vi "log analysis_gps.vi"() -> ()   [LabVIEW 2019] (continued)
\tsystem status\tnormal 2 27.900000 0 0\trobot status\t134.802859\t125.219329\t7.982200\t-2.716402\t-0.059958\t-178.151167\t0.301000\t-0.007000\n\t\n15:45:35.6\tlog_raw\tgps_raw\t#INSPVAXA,USB3,0,48.5,FINESTEERING,2107,283553.600,02000000,471d,15824;INS_ALIGNMENT_COMPLETE,INS_RTKFIXED,37.37125846696,126.72235533990,7.9816,22.3000,0.0235,-0.2652,0.0170,-2.709628745,-0.144831569,268.295218513,0.4383,0.2948,0.5739,0.1125,0.0924,0.0783,0.0963,0.1010,5.0842,0f000001,0*696fd9b1\n\tsystem status\tnormal 2 27.900000 0 0\trobot status\t134.659909\t125.219563\t7.981600\t-2.709629\t-0.144832\t-178.295219\t0.297000\t-0.009000\n\t\n15:45:36.1\tlog_raw\tgps_raw\t#DUALANTENNAHEADINGA,USB3,0,48.5,FINESTEERING,2107,283554.100,02000000,d426,15824;INSUFFICIENT_OBS,NONE,-1.000000000,0.000000000,0.000000000,0.0,0.000000000,0.000000000,\"631T\",13,4,4,3,04,00,20,02*de32c05b\n\tsystem status\tnormal 2 27.900000 0 0\trobot status\t134.520570\t125.219884\t7.981500\t-2.835282\t-0.233687\t-178.487489\t0.302000\t-0.003000\n\t\n15:45:36.6\tlog_raw\tgps_raw\t#INSPVAXA,USB3,0,51.0,FINESTEERING,2107,283554.600,02000000,471d,15824;INS_ALIGNMENT_COMPLETE,INS_RTKFIXED,37.37125848358,126.72235217781,7.9795,22.3000,0.0223,-0.2763,0.0124,-2.892819267,-0.280095971,268.699067349,0.4384,0.2951,0.5740,0.1126,0.0925,0.0783,0.0963,0.1010,5.0853,0f000001,0*82db867f\n\tsystem status\tnormal 2 27.900000 0 0\trobot status\t134.379816\t125.221412\t7.979500\t-2.892819\t-0.280096\t-178.699067\t0.295000\t-0.010000\n\t\n15:45:37.1\tlog_raw\tgps_raw\t#DUALANTENNAHEADINGA,USB3,0,47.0,FINESTEERING,2107,283555.100,02000000,d426,15824;INSUFFICIENT_OBS,NONE,-1.000000000,0.000000000,0.000000000,0.0,0.000000000,0.000000000,\"631T\",14,4,4,3,04,00,20,03*a9c2070c\n\tsystem status\tnormal 2 27.900000 0 0\trobot status\t134.235506\t125.223968\t7.977100\t-2.869099\t-0.294535\t-178.888664\t0.296000\t-0.003000\n\t\n15:45:37.6\tlog_raw\tgps_raw\t#INSPVAXA,USB3,0,47.0,FINESTEERING,2107,283555.600,02000000,471d,15824;INS_ALIGNMENT_COMPLETE,INS_RTKFIXED,37.37125853353,126.72234893237,7.9755,22.3000,0.0216,-0.2860,0.0144,-2.819506648,-0.407770491,269.082070244,0.4381,0.2951,0.5741,0.1126,0.0924,0.0783,0.0963,0.1010,5.0867,0f000001,0*4971d182\n\tsystem status\tnormal 2 27.900000 0 0\trobot status\t134.092341\t125.226961\t7.975500\t-2.819507\t-0.407770\t-179.082070\t0.300000\t-0.010000\n\t\n15:45:38.1\tlog_raw\tgps_raw\t#INSPVAXA,USB3,0,45.0,FINESTEERING,2107,283556.100,02000000,471d,15824;INS_ALIGNMENT_COMPLETE,INS_RTKFIXED,37.37125856914,126.72234737250,7.9744,22.3000,0.0229,-0.2921,0.0135,-2.758204349,-0.398675406,269.289539292,0.4378,0.2952,0.5740,0.1126,0.0924,0.0783,0.0962,0.1010,5.0883,0f000001,0*04f4864c\n\tsystem status\tnormal 2 27.900000 0 0\trobot status\t133.954170\t125.230915\t7.974400\t-2.758204\t-0.398675\t-179.289539\t0.302000\t-0.005000\n\t\n15:45:38.6\tlog_raw\tgps_raw\t#DUALANTENNAHEADINGA,USB3,0,45.0,FINESTEERING,2107,283556.600,02000000,d426,15824;INSUFFICIENT_OBS,NONE,-1.000000000,0.000000000,0.000000000,0.0,0.000000000,0.000000000,\"631T\",14,4,4,3,04,00,20,03*1b8bbdb9\n\tsystem status\tnormal 2 27.900000 0 0\trobot status\t133.810841\t125.235429\t7.973900\t-2.640531\t-0.361099\t-179.438538\t0.158000\t0.018000\n\t\n15:45:39.1\tlog_raw\tgps_raw\t#DUALANTENNAHEADINGA,USB3,0,45.0,FINESTEERING,2107,283557.100,02000000,d426,15824;INSUFFICIENT_OBS,NONE,-1.000000000,0.000000000,0.000000000,0.0,0.000000000,0.000000000,\"631T\",15,4,4,3,04,00,20,03*6d1923ae\n\tsystem status\tnormal 2 27.800000 0 0\trobot status\t133.723563\t125.240390\t7.973200\t-2.680477\t-0.214338\t-179.491663\t0.281000\t-0.012000\n\t\n15:45:39.6\tlog_raw\tgps_raw\t#DUALANTENNAHEADINGA,USB3,0,46.5,FINESTEERING,2107,283557.600,02000000,d426,15824;INSUFFICIENT_OBS,NONE,-1.000000000,0.000000000,0.000000000,0.0,0.000000000,0.000000000,\"631T\",14,4,4,3,04,00,20,03*8fe42440\n\tsystem status\tnormal 2 27.900000 0 0\trobot status\t133.557064\t125.247786\t7.971500\t-2.546712\t-0.382295\t-179.652165\t0.298000\t-0.007000\n\t\n15:45:40.1\tlog_raw\tgps_raw\t#DUALANTENNAHEADINGA,USB3,0,46.5,FINESTEERING,2107,283558.100,02000000,d426,15824;INSUFFICIENT_OBS,NONE,-1.000000000,0.000000000,0.000000000,0.0,0.000000000,0.000000000,\"631T\",11,4,4,3,04,00,20,02*089ab1fe\n\tsystem status\tnormal 2 27.900000 0 0\trobot status\t133.431382\t125.255378\t7.969700\t-2.437296\t-0.317017\t-179.816520\t0.288000\t-0.003000\n\t\n15:45:40.6\tlog_raw\tgps_raw\t#INSPVAXA,USB3,0,47.5,FINESTEERING,2107,283558.600,02000000,471d,15824;INS_ALIGNMENT_COMPLETE,INS_RTKFIXED,37.37125886562,126.72233975708,7.9685,22.3000,0.0526,-0.2759,0.0211,-2.409557071,-0.340107874,269.967780628,0.4378,0.2950,0.5739,0.1125,0.0924,0.0783,0.0962,0.1009,5.0913,0f000001,0*5e667246\n\tsystem status\tnormal 2 27.900000 0 0\trobot status\t133.279608\t125.263831\t7.968500\t-2.409557\t-0.340108\t-179.967781\t0.299000\t0.000000\n\t\n15:45:41.1\tlog_raw\tgps_raw\t#DUALANTENNAHEADINGA,USB3,0,47.5,FINESTEERING,2107,283559.100,02008000,d426,15824;INSUFFICIENT_OBS,NONE,-1.000000000,0.000000000,0.000000000,0.0,0.000000000,0.000000000,\"631T\",9,4,4,3,04,00,20,03*5bfaaf18\n\tsystem status\tnormal 2 27.900000 0 0\trobot status\t133.140609\t125.272278\t7.967700\t-2.441354\t-0.223495\t179.916297\t0.310000\t0.003000\n\t\n15:45:41.6\tlog_raw\tgps_raw\t#DUALANTENNAHEADINGA,USB3,0,51.0,FINESTEERING,2107,283559.600,02008000,d426,15824;INSUFFICIENT_OBS,NONE,-1.000000000,0.000000000,0.000000000,0.0,0.000000000,0.000000000,\"631T\",11,4,4,3,04,00,20,03*aa74f950\n\tsystem status\tnormal 2 27.900000 0 0\trobot status\t132.998565\t125.282342\t7.968400\t-2.323197\t-0.094957\t179.812330\t0.293000\t0.004000\n\t\n15:45:42.1\tlog_raw\tgps_raw\t#DUALANTENNAHEADINGA,USB3,0,43.5,FINESTEERING,2107,283560.100,02008000,d426,15824;INSUFFICIENT_OBS,NONE,-1.000000000,0.000000000,0.000000000,0.0,0.000000000,0.000000000,\"631T\",12,4,4,3,04,00,20,02*918dc314\n\tsystem status\tnormal 2 27.900000 0 0\trobot status\t132.851646\t125.293516\t7.969300\t-2.162737\t0.027270\t179.722426\t0.294000\t0.002000\n\t\n15:45:42.6\tlog_raw\tgps_raw\t#INSPVAXA,USB3,0,43.5,FINESTEERING,2107,283560.600,02008000,471d,15824;INS_ALIGNMENT_COMPLETE,INS_RTKFIXED,37.37125922477,126.72233331539,7.9711,22.3000,0.0461,-0.3029,0.0142,-2.105523961,0.098116504,270.318274292,0.4374,0.2952,0.5740,0.1125,0.0925,0.0783,0.0962,0.1009,5.0942,0f000001,0*4e7a44d6\n\tsystem status\tnormal 2 27.900000 0 0\trobot status\t132.709014\t125.303700\t7.971100\t-2.105524\t0.098117\t179.681726\t0.302000\t0.009000\n\t\n15:45:43.1\tlog_raw\tgps_raw\t\tsystem status\tnormal 2 27.900000 0 0\trobot status\t132.562472\t125.314678\t7.972700\t-2.092784\t0.038712\t179.551571\t0.231000\t0.029000\n\t\n15:45:43.6\tlog_raw\tgps_raw\t#DUALANTENNAHEADINGA,USB3,0,45.0,FINESTEERING,2107,283561.600,02008000,d426,15824;INSUFFICIENT_OBS,NONE,-1.000000000,0.000000000,0.000000000,0.0,0.000000000,0.000000000,\"631T\",11,4,4,3,04,00,20,03*333d7c31\n\tsystem status\tnormal 2 27.800000 0 0\trobot status\t132.438939\t125.326177\t7.973000\t-2.055838\t0.129600\t179.563628\t0.311000\t0.023000\n\t\n15:45:44.1\tlog_raw\tgps_raw\t#DUALANTENNAHEADINGA,USB3,0,45.0,FINESTEERING,2107,283562.100,02008000,d426,15824;INSUFFICIENT_OBS,NONE,-1.000000000,0.000000000,0.000000000,0.0,0.000000000,0.000000000,\"631T\",10,4,4,3,04,00,20,03*9e1feb94\n\tsystem status\tnormal 2 27.900000 0 0\trobot status\t132.286022\t125.338495\t7.973600\t-2.088322\t-0.039362\t179.462499\t0.292000\t0.007000\n\t\n15:45:44.6\tlog_raw\tgps_raw\t#DUALANTENNAHEADINGA,USB3,0,49.5,FINESTEERING,2107,283562.600,02008000,d426,15824;INSUFFICIENT_OBS,NONE,-1.000000000,0.000000000,0.000000000,0.0,0.000000000,0.000000000,\"631T\",11,4,4,3,04,00,20,03*0e8972e5\n\tsystem status\tnormal 2 27.900000 0 0\trobot status\t132.139609\t125.349583\t7.973900\t-2.147199\t-0.245096\t179.550470\t0.291000\t0.030000\n\t\n15:45:45.1\tlog_raw\tgps_raw\t#DUALANTENNAHEADINGA,USB3,0,49.5,FINESTEERING,2107,283563.100,02008000,d426,15824;INSUFFICIENT_OBS,NONE,-1.000000000,0.000000000,0.000000000,0.0,0.000000000,0.000000000,\"631T\",12,4,4,3,04,00,20,03*0cafea03\n\tsystem status\tnormal 2 27.800000 0 0\trobot status\t131.994665\t125.361643\t7.974000\t-2.066885\t-0.502356\t179.731447\t0.253000\t0.073000\n\t\n15:45:45.6\tlog_raw\tgps_raw\t#DUALANTENNAHEADINGA,USB3,0,49.5,FINESTEERING,2107,283563.600,02000000,d426,15824;INSUFFICIENT_OBS,NONE,-1.000000000,0.000000000,0.000000000,0.0,0.000000000,0.000000000,\"631T\",11,4,4,3,04,00,20,03*75c2f29d\n\tsystem status\tnormal 2 27.800000 0 0\trobot status\t131.850322\t125.373668\t7.974200\t-1.867187\t-0.627381\t-179.945539\t0.352000\t-0.066000\n\t\n15:45:46.1\tlog_raw\tgps_raw\t#DUALANTENNAHEADINGA,USB3,0,46.5,FINESTEERING,2107,283564.100,02000000,d426,15824;INSUFFICIENT_OBS,NONE,-1.000000000,0.000000000,0.000000000,0.0,0.000000000,0.000000000,\"631T\",12,4,4,3,04,00,20,03*b22ee873\n\tsystem status\tnormal 2 27.800000 0 0\trobot status\t131.705241\t125.384504\t7.975500\t-1.737840\t-0.783684\t-179.600630\t0.268000\t0.066000\n\t\n15:45:46.6\tlog_raw\tgps_raw\t#DUALANTENNAHEADINGA,USB3,0,46.5,FINESTEERING,2107,283564.600,02000000,d426,15824;INSUFFICIENT_OBS,NONE,-1.000000000,0.000000000,0.000000000,0.0,0.000000000,0.000000000,\"631T\",13,4,4,3,04,00,20,03*a96472bd\n\tsystem status\tnormal 2 27.700000 0 0\trobot status\t131.562793\t125.392691\t7.976300\t-1.793916\t-0.734413\t-179.145443\t0.390000\t-0.097000\n\t\n15:45:47.1\tlog_raw\tgps_raw\t#DUALANTENNAHEADINGA,USB3,0,46.5,FINESTEERING,2107,283565.100,02000000,d426,15824;INSUFFICIENT_OBS,NONE,-1.000000000,0.000000000,0.000000000,0.0,0.000000000,0.000000000,\"631T\",13,4,4,3,04,00,20,03*08146cf2\n\tsystem status\tnormal 2 27.700000 0 0\trobot status\t131.420891\t125.399247\t7.976000\t-1.910475\t-0.662509\t-178.628817\t0.261000\t0.086000\n\t\n15:45:47.6\tlog_raw\tgps_raw\t#DUALANTENNAHEADINGA,USB3,0,48.0,FINESTEERING,2107,283565.600,02000000,d426,15824;INSUFFICIENT_OBS,NONE,-1.000000000,0.000000000,0.000000000,0.0,0.000000000,0.000000000,\"631T\",12,4,4,3,04,00,20,03*500b58cb\n\tsystem status\tnormal 2 27.700000 0 0\trobot status\t131.278267\t125.405143\t7.974600\t-1.874953\t-0.506860\t-178.110215\t0.404000\t-0.126000\n\t\n15:45:48.1\tlog_raw\tgps_raw\t#DUALANTENNAHEADINGA,USB3,0,48.0,FINESTEERING,2107,283566.100,02000000,d426,15824;INSUFFICIENT_OBS,NONE,-1.000000000,0.000000000,0.000000000,0.0,0.000000000,0.000000000,\"631T\",13,4,4,3,04,00,20,02*8a2efff8\n\tsystem status\tnormal 2 27.700000 0 0\trobot status\t131.149443\t125.410077\t7.973900\t-1.835673\t-0.302067\t-177.605096\t0.432000\t-0.159000\n\t\n15:45:48.6\tlog_raw\tgps_raw\t\tsystem status\tnormal 2 27.700000 0 0\trobot status\t131.007001\t125.413685\t7.975600\t-1.683560\t-0.282934\t-177.105716\t0.327000\t-0.010000\n\t\n15:45:49.1\tlog_raw\tgps_raw\t#INSPVAXA,USB3,0,47.0,FINESTEERING,2107,283567.150,02000000,471d,15824;INS_ALIGNMENT_COMPLETE,INS_RTKFIXED,37.37126023924,126.72231232835,7.9766,22.3000,0.0196,-0.2915,0.0203,-1.615683840,-0.184237550,266.738571120,0.4436,0.2960,0.5749,0.1133,0.0925,0.0784,0.0962,0.1011,5.1038,0f000001,0*2b446319\n\tsystem status\tnormal 2 27.700000 0 0\trobot status\t130.850016\t125.416320\t7.976600\t-1.615684\t-0.184238\t-176.738571\t0.310000\t-0.001000\n\t\n15:45:49.6\tlog_raw\tgps_raw\t#DUALANTENNAHEADINGA,USB3,0,47.0,FINESTEERING,2107,283567.600,02000000,d426,15824;INSUFFICIENT_OBS,NONE,-1.000000000,0.000000000,0.000000000,0.0,0.000000000,0.000000000,\"631T\",12,4,4,3,04,00,20,02*8ed7ff70\n\tsystem status\tnormal 2 27.800000 0 0\trobot status\t130.720508\t125.417185\t7.976700\t-1.694653\t-0.119094\t-176.472297\t0.377000\t-0.106000\n\t\n15:45:50.1\tlog_raw\tgps_raw\t#DUALANTENNAHEADINGA,USB3,0,47.0,FINESTEERING,2107,283568.100,02000000,d426,15824;INSUFFICIENT_OBS,NONE,-1.000000000,0.000000000,0.000000000,0.0,0.000000000,0.000000000,\"631T\",14,4,4,3,04,00,20,03*aaffec67\n\tsystem status\tnormal 2 27.800000 0 0\trobot status\t130.578522\t125.417897\t7.977700\t-1.786957\t0.019040\t-176.223413\t0.280000\t0.039000\n\t\n15:45:50.6\tlog_raw\tgps_raw\t#INSPVAXA,USB3,0,50.5,FINESTEERING,2107,283568.650,02000000,471d,15824;INS_ALIGNMENT_COMPLETE,INS_RTKFIXED,37.37126026613,126.72230748127,7.9785,22.3000,0.0314,-0.2890,0.0136,-1.676303872,0.031387209,266.013991723,0.4441,0.2961,0.5750,0.1133,0.0925,0.0784,0.0962,0.1011,5.1051,0f000001,0*382c449f\n\tsystem status\tnormal 2 27.800000 0 0\trobot status\t130.420670\t125.419311\t7.978500\t-1.676304\t0.031387\t-176.013992\t0.335000\t-0.037000\n\t\n15:45:51.1\tlog_raw\tgps_raw\t#DUALANTENNAHEADINGA,USB3,0,40.0,FINESTEERING,2107,283569.100,02000000,d426,15824;INSUFFICIENT_OBS,NONE,-1.000000000,0.000000000,0.000000000,0.0,0.000000000,0.000000000,\"631T\",13,4,4,3,04,00,20,02*1cb1745e\n\tsystem status\tnormal 2 27.800000 0 0\trobot status\t130.289708\t125.420071\t7.978300\t-1.557732\t0.003070\t-175.975563\t0.340000\t-0.063000\n\t\n15:45:51.6\tlog_raw\tgps_raw\t#DUALANTENNAHEADINGA,USB3,0,40.0,FINESTEERING,2107,283569.600,02000000,d426,15824;INSUFFICIENT_OBS,NONE,-1.000000000,0.000000000,0.000000000,0.0,0.000000000,0.000000000,\"631T\",13,4,4,3,04,00,20,03*a71e5e5e\n\tsystem status\tnormal 2 27.800000 0 0\trobot status\t130.146113\t125.419852\t7.978500\t-1.454637\t0.095316\t-175.896222\t0.295000\t0.006000\n\t\n15:45:52.1\tlog_raw\tgps_raw\t#INSPVAXA,USB3,0,51.0,FINESTEERING,2107,283570.150,02000000,471d,15824;INS_ALIGNMENT_COMPLETE,INS_RTKFIXED,37.37126027188,126.72230260848,7.9782,22.3000,0.0223,-0.2985,0.0040,-1.310118648,0.027956781,265.914374243,0.4449,0.2965,0.5753,0.1133,0.0927,0.0784,0.0962,0.1011,5.1080,0f000001,0*e4cc9c92\n\tsystem status\tnormal 2 27.800000 0 0\trobot status\t129.989046\t125.419956\t7.978200\t-1.310119\t0.027957\t-175.914374\t0.293000\t0.021000\n\t\n15:45:52.6\tlog_raw\tgps_raw\t#INSPVAXA,USB3,0,51.0,FINESTEERING,2107,283570.650,02000000,471d,15824;INS_ALIGNMENT_COMPLETE,INS_RTKFIXED,37.37126026750,126.72230111428,7.9776,22.3000,0.0310,-0.1470,0.0080,-1.255276150,-0.174138807,265.875286689,0.4449,0.2965,0.5753,0.1133,0.0927,0.0784,0.0962,0.1011,5.1080,0f000001,0*fb01e8e4\n\tsystem status\tnormal 2 27.900000 0 0\trobot status\t129.856693\t125.419472\t7.977600\t-1.255276\t-0.174139\t-175.875287\t0.139000\t0.065000\n\t\n15:45:53.1\tlog_raw\tgps_raw\t#INSPVAXA,USB3,0,50.0,FINESTEERING,2107,283571.150,02000000,471d,15824;INS_ALIGNMENT_COMPLETE,INS_RTKFIXED,37.37126027111,126.72229951558,7.9776,22.3000,-0.0095,-0.3504,-0.0012,-1.130419534,-0.185484043,265.929537810,0.4449,0.2965,0.5753,0.1133,0.0927,0.0784,0.0962,0.1011,5.1080,0f000001,0*20782363\n\tsystem status\tnormal 2 27.800000 0 0\trobot status\t129.715082\t125.419874\t7.977600\t-1.130420\t-0.185484\t-175.929538\t0.366000\t-0.034000\n\t\n15:45:53.6\tlog_raw\tgps_raw\t\tsystem status\tnormal 2 27.800000 0 0\trobot status\t129.601866\t125.425975\t7.981400\t-0.935962\t-0.226185\t-175.828479\t0.305000\t0.000000\n\t\n15:45:54.1\tlog_raw\tgps_raw\t#DUALANTENNAHEADINGA,USB3,0,50.0,FINESTEERING,2107,283572.100,02000000,d426,15824;INSUFFICIENT_OBS,NONE,0.000000000,0.000000000,0.000000000,0.0,0.000000000,0.000000000,\"\",0,0,0,0,00,00,00,00*5d8535fc\n\tsystem status\tnormal 2 27.900000 0 0\trobot status\t129.452172\t125.430719\t7.986500\t-0.803584\t-0.452987\t-175.991155\t0.278000\t-0.004000\n\t\n15:45:54.6\tlog_raw\tgps_raw\t#DUALANTENNAHEADINGA,USB3,0,52.5,FINESTEERING,2107,283572.600,02000000,d426,15824;INSUFFICIENT_OBS,NONE,0.000000000,0.000000000,0.000000000,0.0,0.000000000,0.000000000,\"\",0,0,0,0,00,00,00,00*859f07a2\n\tsystem status\tnormal 2 27.900000 0 0\trobot status\t129.304513\t125.435695\t7.990800\t-0.754578\t-0.513148\t-176.084037\t0.303000\t-0.001000\n\t\n15:45:55.1\tlog_raw\tgps_raw\t#DUALANTENNAHEADINGA,USB3,0,50.0,FINESTEERING,2107,283573.100,02000000,d426,15824;INSUFFICIENT_OBS,NONE,0.000000000,0.000000000,0.000000000,0.0,0.000000000,0.000000000,\"\",0,0,0,0,00,00,00,00*a797c2ea\n\tsystem status\tnormal 2 27.900000 0 0\trobot status\t129.165268\t125.438398\t7.993900\t-0.825963\t-0.339685\t-176.124396\t0.304000\t0.001000\n\t\n15:45:55.6\tlog_raw\tgps_raw\t\tsystem status\tnormal 2 27.900000 0 0\trobot status\t129.021483\t125.428571\t7.991000\t-0.801949\t-0.273048\t-176.197065\t0.293000\t-0.010000\n\t\n15:45:56.1\tlog_raw\tgps_raw\t\tsystem status\tnormal 2 27.900000 0 0\trobot status\t128.872499\t125.421188\t7.988200\t-0.569716\t-0.162658\t-176.307146\t0.297000\t-0.004000\n\t\n15:45:56.6\tlog_raw\tgps_raw\t#INSPVAXA,USB3,0,52.0,FINESTEERING,2107,283574.650,02000000,471d,15824;INS_ALIGNMENT_COMPLETE,INS_RTKFIXED,37.37126025479,126.72228822591,7.9861,22.3000,0.0090,-0.3026,-0.0003,-0.524199220,-0.126443269,266.389234836,0.4991,0.3317,0.6500,0.1205,0.0986,0.0804,0.0985,0.1030,5.1132,0f000001,0*c3c99d89\n\tsystem status\tnormal 2 27.900000 0 0\trobot status\t128.715062\t125.418079\t7.986100\t-0.524199\t-0.126443\t-176.389235\t0.303000\t-0.004000\n\t\n15:45:57.1\tlog_raw\tgps_raw\t#INSPVAXA,USB3,0,50.0,FINESTEERING,2107,283575.150,02000000,471d,15824;INS_ALIGNMENT_COMPLETE,INS_RTKFIXED,37.37126023129,126.72228662486,7.9852,22.3000,0.0085,-0.2932,0.0017,-0.596688743,-0.097225443,266.485321234,0.4751,0.3142,0.6322,0.1185,0.0977,0.0789,0.0982,0.1027,5.1147,0f000001,0*e174b094\n\tsystem status\tnormal 2 27.900000 0 0\trobot status\t128.573243\t125.415473\t7.985200\t-0.596689\t-0.097225\t-176.485321\t0.297000\t-0.011000\n\t\n15:45:57.6\tlog_raw\tgps_raw\t#INSPVAXA,USB3,0,50.0,FINESTEERING,2107,283575.650,02000000,471d,15824;INS_ALIGNMENT_COMPLETE,INS_RTKFIXED,37.37126022571,126.72228518067,7.9842,22.3000,-0.0010,-0.2887,0.0210,-0.683424263,-0.147084143,266.527685008,0.4751,0.3142,0.6322,0.1185,0.0977,0.0789,0.0982,0.1027,5.1147,0f000001,0*c2e268d1\n\tsystem status\tnormal 2 27.900000 0 0\trobot status\t128.445319\t125.414855\t7.984200\t-0.683424\t-0.147084\t-176.527685\t0.295000\t-0.014000\n\t\n15:45:58.1\tlog_raw\tgps_raw\t#INSPVAXA,USB3,0,50.0,FINESTEERING,2107,283576.150,02000000,471d,15824;INS_ALIGNMENT_COMPLETE,INS_RTKFIXED,37.37126021633,126.72228346240,7.9840,22.3000,0.0021,-0.2751,0.0114,-0.667866815,-0.315367181,266.708831075,0.4606,0.3053,0.6179,0.1181,0.0979,0.0781,0.0979,0.1024,5.1163,0f000001,0*0ba78e3d\n\tsystem status\tnormal 2 27.900000 0 0\trobot status\t128.293118\t125.413817\t7.984000\t-0.667867\t-0.315367\t-176.708831\t0.298000\t-0.010000\n\t\n15:45:58.6\tlog_raw\tgps_raw\t#INSPVAXA,USB3,0,50.0,FINESTEERING,2107,283576.650,02000000,471d,15824;INS_ALIGNMENT_COMPLETE,INS_RTKFIXED,37.37126022512,126.72228190722,7.9848,22.3000,-0.0006,-0.2994,0.0229,-0.670999350,-0.155338039,266.786409078,0.4606,0.3053,0.6179,0.1181,0.0979,0.0781,0.0979,0.1024,5.1163,0f000001,0*9811c325\n\tsystem status\tnormal 2 27.900000 0 0\trobot status\t128.155363\t125.414794\t7.984800\t-0.670999\t-0.155338\t-176.786409\t0.310000\t-0.008000\n\t\n15:45:59.1\tlog_raw\tgps_raw\t\tsystem status\tnormal 2 27.900000 0 0\trobot status\t128.030138\t125.416182\t7.985200\t-0.637257\t-0.102027\t-176.886811\t0.297000\t-0.010000\n\t\n15:45:59.6\tlog_raw\tgps_raw\t#INSPVAXA,USB3,0,48.5,FINESTEERING,2107,283577.650,02000000,471d,15824;INS_ALIGNMENT_COMPLETE,INS_RTKFIXED,37.37126026454,126.72227868899,7.9856,22.3000,0.0080,-0.2785,0.0173,-0.609374053,-0.154098562,267.060666338,0.4521,0.3012,0.6064,0.1181,0.0980,0.0776,0.0975,0.1023,5.1178,0f000001,0*aa9c2bc5\n\tsystem status\tnormal 2 27.900000 0 0\trobot status\t127.870297\t125.419174\t7.985600\t-0.609374\t-0.154099\t-177.060666\t0.297000\t-0.010000\n\t\n15:46:00.1\tlog_raw\tgps_raw\t\tsystem status\tnormal 2 27.900000 0 0\trobot status\t127.740454\t125.423243\t7.986100\t-0.487780\t-0.129325\t-177.210178\t0.305000\t-0.013000\n\t\n15:46:00.6\tlog_raw\tgps_raw\t\tsystem status\tnormal 2 27.900000 0 0\trobot status\t127.598271\t125.426877\t7.987900\t-0.577346\t-0.157853\t-177.428203\t0.301000\t-0.011000\n\t\n15:46:01.1\tlog_raw\tgps_raw\t#INSPVAXA,USB3,0,51.5,FINESTEERING,2107,283579.150,02000000,471d,15824;INS_ALIGNMENT_COMPLETE,INS_RTKFIXED,37.37126037410,126.72227378516,7.9904,22.3000,0.0163,-0.2830,0.0173,-0.746603441,-0.380752059,267.626447850,0.4463,0.2992,0.5904,0.1180,0.0971,0.0775,0.0966,0.1018,5.1209,0f000001,0*da9a51df\n\tsystem status\tnormal 2 27.900000 0 0\trobot status\t127.435924\t125.431340\t7.990400\t-0.746603\t-0.380752\t-177.626448\t0.295000\t0.002000\n\t\n15:46:01.6\tlog_raw\tgps_raw\t#INSPVAXA,USB3,0,51.5,FINESTEERING,2107,283579.650,02000000,471d,15824;INS_ALIGNMENT_COMPLETE,INS_RTKFIXED,37.37126042399,126.72227213267,7.9925,22.3000,0.0129,-0.2940,0.0192,-0.723337751,-0.333271037,267.787526970,0.4463,0.2992,0.5904,0.1180,0.0971,0.0775,0.0966,0.1018,5.1209,0f000001,0*2d4308ff\n\tsystem status\tnormal 2 27.900000 0 0\trobot status\t127.289549\t125.436879\t7.992500\t-0.723338\t-0.333271\t-177.787527\t0.298000\t-0.005000\n\t\n15:46:02.1\tlog_raw\tgps_raw\t#INSPVAXA,USB3,0,52.5,FINESTEERING,2107,283580.150,02000000,471d,15824;INS_ALIGNMENT_COMPLETE,INS_RTKFIXED,37.37126049043,126.72227055501,7.9950,22.3000,0.0243,-0.3033,0.0180,-0.573377117,-0.330323438,267.951447700,0.4448,0.2989,0.5852,0.1175,0.0961,0.0776,0.0961,0.1014,5.1224,0f000001,0*65285ec1\n\tsystem status\tnormal 2 27.900000 0 0\trobot status\t127.149802\t125.444255\t7.995000\t-0.573377\t-0.330323\t-177.951448\t0.300000\t-0.003000\n\t\n15:46:02.6\tlog_raw\tgps_raw\t\tsystem status\tnormal 2 27.900000 0 0\trobot status\t127.021740\t125.451168\t7.997000\t-0.486595\t-0.381728\t-178.092435\t0.295000\t-0.004000\n\t\n15:46:03.1\tlog_raw\tgps_raw\t#DUALANTENNAHEADINGA,USB3,0,48.0,FINESTEERING,2107,283581.100,02000000,d426,15824;INSUFFICIENT_OBS,NONE,0.000000000,0.000000000,0.000000000,0.0,0.000000000,0.000000000,\"\",0,0,0,0,00,00,00,00*0d472a41\n\tsystem status\tnormal 2 27.900000 0 0\trobot status\t126.878207\t125.458703\t7.999100\t-0.601198\t-0.320020\t-178.256056\t0.297000\t0.000000\n\t\n15:46:03.6\tlog_raw\tgps_raw\t#INSPVAXA,USB3,0,48.0,FINESTEERING,2107,283581.650,02000000,471d,15824;INS_ALIGNMENT_COMPLETE,INS_RTKFIXED,37.37126070396,126.72226577509,8.0028,22.3000,0.0230,-0.2933,0.0344,-0.578760971,-0.170041590,268.380757067,0.4441,0.2986,0.5812,0.1168,0.0951,0.0777,0.0958,0.1011,5.1238,0f000001,0*94c5c4b2\n\tsystem status\tnormal 2 27.900000 0 0\trobot status\t126.726405\t125.467960\t8.002800\t-0.578761\t-0.170042\t-178.380757\t0.306000\t-0.001000\n\t\n15:46:04.1\tlog_raw\tgps_raw\t\tsystem status\tnormal 2 27.900000 0 0\trobot status\t126.600259\t125.475820\t8.006300\t-0.540708\t-0.165891\t-178.462661\t0.304000\t0.009000\n\t\n15:46:04.6\tlog_raw\tgps_raw\t#INSPVAXA,USB3,0,50.0,FINESTEERING,2107,283582.650,02000000,471d,15824;INS_ALIGNMENT_COMPLETE,INS_RTKFIXED,37.37126086300,126.72226255094,8.0114,22.3000,0.0186,-0.2902,0.0297,-0.554451124,-0.113657827,268.567093928,0.4437,0.2982,0.5783,0.1160,0.0941,0.0779,0.0956,0.1009,5.1252,0f000001,0*de1d38ac\n\tsystem status\tnormal 2 27.900000 0 0\trobot status\t126.440815\t125.485615\t8.011400\t-0.554451\t-0.113658\t-178.567094\t0.299000\t0.008000\n\t\n15:46:05.1\tlog_raw\tgps_raw\t#INSPVAXA,USB3,0,52.0,FINESTEERING,2107,283583.150,02000000,471d,15824;INS_ALIGNMENT_COMPLETE,INS_RTKFIXED,37.37126094107,126.72226089314,8.0147,22.3000,0.0176,-0.2816,0.0224,-0.681553326,-0.108375043,268.657687253,0.4431,0.2976,0.5763,0.1151,0.0933,0.0781,0.0955,0.1007,5.1266,0f000001,0*8a630b8d\n\tsystem status\tnormal 2 27.900000 0 0\trobot status\t126.293970\t125.494282\t8.014700\t-0.681553\t-0.108375\t-178.657687\t0.297000\t0.007000\n\t\n15:46:05.6\tlog_raw\tgps_raw\t#INSPVAXA,USB3,0,52.0,FINESTEERING,2107,283583.650,02000000,471d,15824;INS_ALIGNMENT_COMPLETE,INS_RTKFIXED,37.37126102705,126.72225926038,8.0174,22.3000,0.0194,-0.3033,0.0147,-0.616207417,-0.286762817,268.672715403,0.4431,0.2976,0.5763,0.1151,0.0933,0.0781,0.0955,0.1007,5.1266,0f000001,0*61848793\n\tsystem status\tnormal 2 27.900000 0 0\trobot status\t126.149343\t125.503827\t8.017400\t-0.616207\t-0.286763\t-178.672715\t0.308000\t0.006000\n\t\n15:46:06.1\tlog_raw\tgps_raw\t#INSPVAXA,USB3,0,52.0,FINESTEERING,2107,283584.150,02000000,471d,15824;INS_ALIGNMENT_COMPLETE,INS_RTKFIXED,37.37126112105,126.72225762489,8.0208,22.3000,0.0251,-0.2868,0.0143,-0.484996115,-0.348090113,268.682050647,0.4426,0.2969,0.5750,0.1144,0.0927,0.0782,0.0955,0.1006,5.1279,0f000001,0*d30f3e54\n\tsystem status\tnormal 2 27.900000 0 0\trobot status\t126.004474\t125.514261\t8.020800\t-0.484996\t-0.348090\t-178.682051\t0.301000\t0.006000\n\t\n15:46:06.6\tlog_raw\tgps_raw\t#INSPVAXA,USB3,0,52.0,FINESTEERING,2107,283584.650,02000000,471d,15824;INS_ALIGNMENT_COMPLETE,INS_RTKFIXED,37.37126121621,126.72225620166,8.0227,22.3000,0.0321,-0.0816,0.0199,-0.459149355,-0.498683965,268.628376377,0.4426,0.2969,0.5750,0.1144,0.0927,0.0782,0.0955,0.1006,5.1279,0f000001,0*e5ed7c63\n\tsystem status\tnormal 2 27.900000 0 0\trobot status\t125.878406\t125.524825\t8.022700\t-0.459149\t-0.498684\t-178.628376\t0.142000\t0.011000\n\t\n15:46:07.1\tlog_raw\tgps_raw\t#INSPVAXA,USB3,0,49.0,FINESTEERING,2107,283585.150,02000000,471d,15824;INS_ALIGNMENT_COMPLETE,INS_RTKFIXED,37.37126129698,126.72225459849,8.0251,22.3000,0.0349,-0.3426,0.0329,-0.569349800,-0.560640511,268.532383253,0.4425,0.2966,0.5744,0.1144,0.0924,0.0784,0.0956,0.1006,5.1294,0f000001,0*4640cbf6\n\tsystem status\tnormal 2 27.700000 0 0\trobot status\t125.736400\t125.533791\t8.025100\t-0.569350\t-0.560641\t-178.532383\t0.389000\t-0.081000\n\t\n15:46:07.6\tlog_raw\tgps_raw\t#INSPVAXA,USB3,0,49.0,FINESTEERING,2107,283585.650,02000000,471d,15824;INS_ALIGNMENT_COMPLETE,INS_RTKFIXED,37.37126137394,126.72225308543,8.0277,22.3000,0.0305,-0.3477,0.0168,-0.707352535,-0.516144165,268.333596331,0.4425,0.2966,0.5744,0.1144,0.0924,0.0784,0.0956,0.1006,5.1294,0f000001,0*ea5ffab2\n\tsystem status\tnormal 2 27.800000 0 0\trobot status\t125.602376\t125.542334\t8.027700\t-0.707353\t-0.516144\t-178.333596\t0.335000\t0.002000\n\t\n15:46:08.1\tlog_raw\tgps_raw\t#INSPVAXA,USB3,0,50.5,FINESTEERING,2107,283586.150,02000000,471d,15824;INS_ALIGNMENT_COMPLETE,INS_RTKFIXED,37.37126146482,126.72225147889,8.0290,22.3000,0.0318,-0.3117,0.0162,-0.540726540,-0.516678625,268.023762114,0.4406,0.2960,0.5741,0.1134,0.0922,0.0785,0.0957,0.1006,5.1306,0f000001,0*2ae37417\n\tsystem status\tnormal 2 27.800000 0 0\trobot status\t125.460071\t125.552423\t8.029000\t-0.540727\t-0.516679\t-178.023762\t0.289000\t0.030000\n\t\n15:46:08.6\tlog_raw\tgps_raw\t#INSPVAXA,USB3,0,50.5,FINESTEERING,2107,283586.650,02000000,471d,15824;INS_ALIGNMENT_COMPLETE,INS_RTKFIXED,37.37126154442,126.72224983237,8.0302,22.3000,0.0153,-0.2976,0.0132,-0.405221817,-0.801510438,267.749524136,0.4406,0.2960,0.5741,0.1134,0.0922,0.0785,0.0957,0.1006,5.1306,0f000001,0*889b905c\n\tsystem status\tnormal 2 27.800000 0 0\trobot status\t125.314225\t125.561259\t8.030200\t-0.405222\t-0.801510\t-177.749524\t0.329000\t-0.031000\n\t\n15:46:09.1\tlog_raw\tgps_raw\t#INSPVAXA,USB3,0,48.5,FINESTEERING,2107,283587.150,02000000,471d,15824;INS_ALIGNMENT_COMPLETE,INS_RTKFIXED,37.37126161078,126.72224818389,8.0314,22.3000,0.0135,-0.2861,0.0058,-0.357423684,-1.016170306,267.360005702,0.4401,0.2956,0.5740,0.1128,0.0921,0.0786,0.0958,0.1006,5.1321,0f000001,0*b354eb89\n\tsystem status\tnormal 2 27.700000 0 0\trobot status\t125.168205\t125.568626\t8.031400\t-0.357424\t-1.016170\t-177.360006\t0.215000\t0.133000\n\t\n15:46:09.6\tlog_raw\tgps_raw\t#DUALANTENNAHEADINGA,USB3,0,48.5,FINESTEERING,2107,283587.600,02000000,d426,15824;INSUFFICIENT_OBS,NONE,0.000000000,0.000000000,0.000000000,0.0,0.000000000,0.000000000,\"\",0,0,0,0,00,00,00,00*3e024a6f\n\tsystem status\tnormal 2 27.700000 0 0\trobot status\t125.039123\t125.573448\t8.032800\t-0.358744\t-1.223027\t-176.913005\t0.232000\t0.115000\n\t\n15:46:10.1\tlog_raw\tgps_raw\t\tsystem status\tnormal 2 27.700000 0 0\trobot status\t124.894346\t125.578707\t8.033000\t-0.333259\t-1.304373\t-176.475504\t0.206000\t0.158000\n\t\n15:46:10.6\tlog_raw\tgps_raw\t#INSPVAXA,USB3,0,49.5,FINESTEERING,2107,283588.650,02000000,471d,15824;INS_ALIGNMENT_COMPLETE,INS_RTKFIXED,37.37126174157,126.72224330005,8.0321,22.3000,0.0403,-0.2838,0.0098,-0.134470490,-1.230467800,265.991496419,0.4395,0.2955,0.5741,0.1126,0.0921,0.0786,0.0959,0.1007,5.1336,0f000001,0*86c47da8\n\tsystem status\tnormal 2 27.700000 0 0\trobot status\t124.735603\t125.583149\t8.032100\t-0.134470\t-1.230468\t-175.991496\t0.276000\t0.046000\n\t\n15:46:11.1\tlog_raw\tgps_raw\t#INSPVAXA,USB3,0,51.5,FINESTEERING,2107,283589.150,02000000,471d,15824;INS_ALIGNMENT_COMPLETE,INS_RTKFIXED,37.37126177483,126.72224169465,8.0328,22.3000,0.0428,-0.2922,0.0200,-0.044724950,-0.991745549,265.567471181,0.4384,0.2954,0.5742,0.1124,0.0922,0.0786,0.0960,0.1008,5.1352,0f000001,0*fd2974d4\n\tsystem status\tnormal 2 27.700000 0 0\trobot status\t124.593399\t125.586842\t8.032800\t-0.044725\t-0.991746\t-175.567471\t0.295000\t0.021000\n\t\n15:46:11.6\tlog_raw\tgps_raw\t#INSPVAXA,USB3,0,51.5,FINESTEERING,2107,283589.650,02000000,471d,15824;INS_ALIGNMENT_COMPLETE,INS_RTKFIXED,37.37126179570,126.72224014857,8.0325,22.3000,0.0430,-0.3072,0.0249,-0.007617366,-0.680507333,265.196792969,0.4384,0.2954,0.5742,0.1124,0.0922,0.0786,0.0960,0.1008,5.1352,0f000001,0*75474069\n\tsystem status\tnormal 2 27.700000 0 0\trobot status\t124.456450\t125.589160\t8.032500\t-0.007617\t-0.680507\t-175.196793\t0.366000\t-0.059000\n\t\n15:46:12.1\tlog_raw\tgps_raw\t#INSPVAXA,USB3,0,52.0,FINESTEERING,2107,283590.150,02000000,471d,15824;INS_ALIGNMENT_COMPLETE,INS_RTKFIXED,37.37126181306,126.72223852203,8.0321,22.3000,0.0371,-0.3064,0.0221,-0.054866167,-0.319461022,264.939008114,0.4379,0.2954,0.5744,0.1124,0.0922,0.0786,0.0960,0.1008,5.1368,0f000001,0*489db8a8\n\tsystem status\tnormal 2 27.800000 0 0\trobot status\t124.312374\t125.591089\t8.032100\t-0.054866\t-0.319461\t-174.939008\t0.268000\t0.071000\n\t\n15:46:12.6\tlog_raw\tgps_raw\t#INSPVAXA,USB3,0,52.0,FINESTEERING,2107,283590.650,02000000,471d,15824;INS_ALIGNMENT_COMPLETE,INS_RTKFIXED,37.37126182845,126.72223689511,8.0304,22.3000,0.0329,-0.2983,0.0263,-0.099615260,-0.144209123,264.670119268,0.4379,0.2954,0.5744,0.1124,0.0922,0.0786,0.0960,0.1008,5.1368,0f000001,0*3ff0cb58\n\tsystem status\tnormal 2 27.800000 0 0\trobot status\t124.168264\t125.592799\t8.030400\t-0.099615\t-0.144209\t-174.670119\t0.312000\t-0.012000\n\t\n15:46:13.1\tlog_raw\tgps_raw\t\tsystem status\tnormal 2 27.800000 0 0\trobot status\t124.023646\t125.595225\t8.029500\t-0.060509\t-0.092324\t-174.506927\t0.241000\t0.080000\n\t\n15:46:13.6\tlog_raw\tgps_raw\t#INSPVAXA,USB3,0,46.5,FINESTEERING,2107,283591.650,02000000,471d,15824;INS_ALIGNMENT_COMPLETE,INS_RTKFIXED,37.37126184009,126.72223359143,8.0280,22.3000,0.0242,-0.3040,0.0144,-0.139661559,-0.269205347,264.433455917,0.4387,0.2955,0.5748,0.1127,0.0923,0.0786,0.0961,0.1009,5.1382,0f000001,0*bb357185\n\tsystem status\tnormal 2 27.800000 0 0\trobot status\t123.875629\t125.594096\t8.028000\t-0.139662\t-0.269205\t-174.433456\t0.245000\t0.087000\n\t\n15:46:14.1\tlog_raw\tgps_raw\t#INSPVAXA,USB3,0,50.0,FINESTEERING,2107,283592.150,02000000,471d,15824;INS_ALIGNMENT_COMPLETE,INS_RTKFIXED,37.37126183340,126.72223190361,8.0268,22.3000,0.0217,-0.3070,0.0246,-0.250767704,-0.520528814,264.430385141,0.4392,0.2956,0.5751,0.1125,0.0924,0.0786,0.0961,0.1010,5.1393,0f000001,0*012bab97\n\tsystem status\tnormal 2 27.800000 0 0\trobot status\t123.726125\t125.593355\t8.026800\t-0.250768\t-0.520529\t-174.430385\t0.403000\t-0.156000\n\t\n15:46:14.6\tlog_raw\tgps_raw\t#INSPVAXA,USB3,0,50.0,FINESTEERING,2107,283592.650,02000000,471d,15824;INS_ALIGNMENT_COMPLETE,INS_RTKFIXED,37.37126182669,126.72223026122,8.0254,22.3000,0.0249,-0.2956,0.0206,-0.309442980,-0.761179345,264.440443486,0.4392,0.2956,0.5751,0.1125,0.0924,0.0786,0.0961,0.1010,5.1393,0f000001,0*78c848e1\n\tsystem status\tnormal 2 27.800000 0 0\trobot status\t123.580645\t125.592613\t8.025400\t-0.309443\t-0.761179\t-174.440443\t0.285000\t0.009000\n\t\n15:46:15.1\tlog_raw\tgps_raw\t\tsystem status\tnormal 2 27.900000 0 0\trobot status\t123.432902\t125.591557\t8.023600\t-0.380611\t-1.050577\t-174.478362\t0.260000\t0.051000\n\t\n15:46:15.6\tlog_raw\tgps_raw\t#INSPVAXA,USB3,0,44.5,FINESTEERING,2107,283593.650,02000000,471d,15824;INS_ALIGNMENT_COMPLETE,INS_RTKFIXED,37.37126179813,126.72222695533,8.0221,22.3000,0.0365,-0.2965,0.0185,-0.369051929,-1.148324870,264.580362201,0.4393,0.2956,0.5754,0.1125,0.0925,0.0786,0.0962,0.1010,5.1403,0f000001,0*8be4a412\n\tsystem status\tnormal 2 27.900000 0 0\trobot status\t123.287814\t125.589447\t8.022100\t-0.369052\t-1.148325\t-174.580362\t0.301000\t-0.019000\n\t\n15:46:16.1\tlog_raw\tgps_raw\t#INSPVAXA,USB3,0,43.0,FINESTEERING,2107,283594.150,02000000,471d,15824;INS_ALIGNMENT_COMPLETE,INS_RTKFIXED,37.37126178881,126.72222531638,8.0209,22.3000,0.0318,-0.2892,0.0117,-0.315197782,-1.127826299,264.669850736,0.4395,0.2956,0.5757,0.1126,0.0925,0.0786,0.0962,0.1010,5.1415,0f000001,0*2d917e72\n\tsystem status\tnormal 2 27.900000 0 0\trobot status\t123.142639\t125.588415\t8.020900\t-0.315198\t-1.127826\t-174.669851\t0.293000\t-0.008000\n\t\n15:46:16.6\tlog_raw\tgps_raw\t#INSPVAXA,USB3,0,43.0,FINESTEERING,2107,283594.650,02000000,471d,15824;INS_ALIGNMENT_COMPLETE,INS_RTKFIXED,37.37126177423,126.72222371508,8.0192,22.3000,0.0303,-0.3062,0.0087,-0.244943668,-0.998392292,264.739545635,0.4395,0.2956,0.5757,0.1126,0.0925,0.0786,0.0962,0.1010,5.1415,0f000001,0*36684632\n\tsystem status\tnormal 2 27.900000 0 0\trobot status\t123.000798\t125.586799\t8.019200\t-0.244944\t-0.998392\t-174.739546\t0.301000\t-0.009000\n\t\n15:46:17.1\tlog_raw\tgps_raw\t#INSPVAXA,USB3,0,48.0,FINESTEERING,2107,283595.150,02000000,471d,15824;INS_ALIGNMENT_COMPLETE,INS_RTKFIXED,37.37126177448,126.72222209651,8.0178,22.3000,0.0339,-0.2977,0.0111,-0.119926645,-0.839441888,264.806746859,0.4396,0.2957,0.5758,0.1127,0.0925,0.0786,0.0962,0.1011,5.1428,0f000001,0*08adb1ac\n\tsystem status\tnormal 2 27.900000 0 0\trobot status\t122.857428\t125.586829\t8.017800\t-0.119927\t-0.839442\t-174.806747\t0.293000\t-0.006000\n\t\n15:46:17.6\tlog_raw\tgps_raw\t#INSPVAXA,USB3,0,48.0,FINESTEERING,2107,283595.650,02000000,471d,15824;INS_ALIGNMENT_COMPLETE,INS_RTKFIXED,37.37126175579,126.72222044305,8.0158,22.3000,0.0315,-0.2901,0.0146,-0.140682450,-0.757275423,264.939327324,0.4396,0.2957,0.5758,0.1127,0.0925,0.0786,0.0962,0.1011,5.1428,0f000001,0*78aa4323\n\tsystem status\tnormal 2 27.900000 0 0\trobot status\t122.710967\t125.584757\t8.015800\t-0.140682\t-0.757275\t-174.939327\t0.293000\t-0.013000\n\t\n15:46:18.1\tlog_raw\tgps_raw\t#INSPVAXA,USB3,0,45.5,FINESTEERING,2107,283596.150,02000000,471d,15824;INS_ALIGNMENT_COMPLETE,INS_RTKFIXED,37.37126174706,126.72221882268,8.0135,22.3000,0.0328,-0.3087,0.0055,-0.159363223,-0.689273148,265.030991748,0.4393,0.2956,0.5759,0.1126,0.0925,0.0785,0.0962,0.1010,5.1440,0f000001,0*bc7a17e4\n\tsystem status\tnormal 2 27.900000 0 0\trobot status\t122.567437\t125.583790\t8.013500\t-0.159363\t-0.689273\t-175.030992\t0.303000\t-0.003000\n\t\n15:46:18.6\tlog_raw\tgps_raw\t\tsystem status\tnormal 2 27.900000 0 0\trobot status\t122.443057\t125.582942\t8.010900\t-0.183483\t-0.673980\t-175.113235\t0.294000\t-0.012000\n\t\n15:46:19.1\tlog_raw\tgps_raw\t\tsystem status\tnormal 2 27.900000 0 0\trobot status\t122.281661\t125.583359\t8.007500\t-0.023917\t-0.662061\t-175.270365\t0.293000\t-0.012000\n\t\n15:46:19.6\tlog_raw\tgps_raw\t#INSPVAXA,USB3,0,47.0,FINESTEERING,2107,283597.650,02000000,471d,15824;INS_ALIGNMENT_COMPLETE,INS_RTKFIXED,37.37126174585,126.72221399388,8.0051,22.3000,0.0336,-0.3137,-0.0021,0.019465738,-0.716944354,265.373596079,0.4393,0.2957,0.5759,0.1127,0.0925,0.0785,0.0962,0.1010,5.1453,0f000001,0*fd9fbe4c\n\tsystem status\tnormal 2 27.900000 0 0\trobot status\t122.139710\t125.583662\t8.005100\t0.019466\t-0.716944\t-175.373596\t0.301000\t-0.008000\n\t\n15:46:20.1\tlog_raw\tgps_raw\t#INSPVAXA,USB3,0,50.5,FINESTEERING,2107,283598.150,02000000,471d,15824;INS_ALIGNMENT_COMPLETE,INS_RTKFIXED,37.37126175152,126.72221241027,8.0034,22.3000,0.0326,-0.3115,-0.0006,-0.014551220,-0.589641139,265.465982891,0.4393,0.2958,0.5760,0.1127,0.0925,0.0785,0.0962,0.1010,5.1467,0f000001,0*f52d235f\n\tsystem status\tnormal 2 27.900000 0 0\trobot status\t121.999437\t125.584293\t8.003400\t-0.014551\t-0.589641\t-175.465983\t0.302000\t-0.013000\n\t\n15:46:20.6\tlog_raw\tgps_raw\t#INSPVAXA,USB3,0,50.5,FINESTEERING,2107,283598.650,02000000,471d,15824;INS_ALIGNMENT_COMPLETE,INS_RTKFIXED,37.37126174603,126.72221081507,8.0012,22.3000,0.0404,-0.2514,0.0050,0.007312732,-0.531763508,265.590138557,0.4393,0.2958,0.5760,0.1127,0.0925,0.0785,0.0962,0.1010,5.1467,0f000001,0*8824c4d8\n\tsystem status\tnormal 2 27.900000 0 0\trobot status\t121.858136\t125.583686\t8.001200\t0.007313\t-0.531764\t-175.590139\t0.233000\t-0.016000\n\t\n15:46:21.1\tlog_raw\tgps_raw\t#INSPVAXA,USB3,0,47.5,FINESTEERING,2107,283599.150,02000000,471d,15824;INS_ALIGNMENT_COMPLETE,INS_RTKFIXED,37.37126176062,126.72220950725,7.9992,22.3000,0.0252,-0.3434,0.0010,0.008395245,-0.454774563,265.666808103,0.4392,0.2959,0.5760,0.1129,0.0925,0.0784,0.0962,0.1010,5.1480,0f000001,0*d239d7e1\n\tsystem status\tnormal 2 27.800000 0 0\trobot status\t121.742292\t125.585307\t7.999200\t0.008395\t-0.454775\t-175.666808\t0.310000\t-0.006000\n\t\n15:46:21.6\tlog_raw\tgps_raw\t\tsystem status\tnormal 2 27.900000 0 0\trobot status\t121.595857\t125.583960\t7.996800\t0.150310\t-0.459246\t-175.818392\t0.292000\t-0.006000\n\t\n15:46:22.1\tlog_raw\tgps_raw\t#INSPVAXA,USB3,0,49.0,FINESTEERING,2107,283600.150,02000000,471d,15824;INS_ALIGNMENT_COMPLETE,INS_RTKFIXED,37.37126175398,126.72220624813,7.9941,22.3000,0.0263,-0.2975,0.0106,0.196462892,-0.509026578,265.990503300,0.4393,0.2959,0.5760,0.1126,0.0926,0.0784,0.0962,0.1010,5.1489,0f000001,0*3b9f52b7\n\tsystem status\tnormal 2 27.900000 0 0\trobot status\t121.453604\t125.584574\t7.994100\t0.196463\t-0.509027\t-175.990503\t0.299000\t-0.007000\n\t\n15:46:22.6\tlog_raw\tgps_raw\t\tsystem status\tnormal 2 27.900000 0 0\trobot status\t121.309342\t125.584758\t7.991000\t0.127952\t-0.446186\t-176.155378\t0.300000\t-0.007000\n\t\n15:46:23.1\tlog_raw\tgps_raw\t#INSPVAXA,USB3,0,49.0,FINESTEERING,2107,283601.150,02000000,471d,15824;INS_ALIGNMENT_COMPLETE,INS_RTKFIXED,37.37126176703,126.72220301301,7.9883,22.3000,0.0322,-0.3028,0.0049,0.082285729,-0.304157914,266.276129441,0.4386,0.2961,0.5760,0.1125,0.0925,0.0784,0.0962,0.1009,5.1498,0f000001,0*cfc5bf1f\n\tsystem status\tnormal 2 27.900000 0 0\trobot status\t121.167043\t125.586027\t7.988300\t0.082286\t-0.304158\t-176.276129\t0.307000\t-0.008000\n\t\n15:46:23.6\tlog_raw\tgps_raw\t#INSPVAXA,USB3,0,49.0,FINESTEERING,2107,283601.650,02000000,471d,15824;INS_ALIGNMENT_COMPLETE,INS_RTKFIXED,37.37126177893,126.72220143158,7.9847,22.3000,0.0347,-0.3053,0.0090,0.167695581,-0.286452712,266.390208904,0.4386,0.2961,0.5760,0.1125,0.0925,0.0784,0.0962,0.1009,5.1498,0f000001,0*1c01ffd1\n\tsystem status\tnormal 2 27.900000 0 0\trobot status\t121.026962\t125.587349\t7.984700\t0.167696\t-0.286453\t-176.390209\t0.301000\t-0.009000\n\t\n15:46:24.1\tlog_raw\tgps_raw\t#INSPVAXA,USB3,0,50.0,FINESTEERING,2107,283602.150,02000000,471d,15824;INS_ALIGNMENT_COMPLETE,INS_RTKFIXED,37.37126180222,126.72219979604,7.9806,22.3000,0.0339,-0.2918,-0.0010,0.296365252,-0.279449744,266.507882837,0.4383,0.2960,0.5760,0.1125,0.0926,0.0784,0.0962,0.1009,5.1509,0f000001,0*8cd233aa\n\tsystem status\tnormal 2 27.900000 0 0\trobot status\t120.882089\t125.589936\t7.980600\t0.296365\t-0.279450\t-176.507883\t0.297000\t-0.003000\n\t\n15:46:24.6\tlog_raw\tgps_raw\t\tsystem status\tnormal 2 27.900000 0 0\trobot status\t120.737723\t125.591847\t7.976700\t0.384711\t-0.490867\t-176.649266\t0.303000\t-0.006000\n\t\n15:46:25.1\tlog_raw\tgps_raw\t\tsystem status\tnormal 2 27.900000 0 0\trobot status\t120.595720\t125.594991\t7.974400\t0.325797\t-0.740098\t-176.797664\t0.272000\t0.005000\n\t\n15:46:25.6\tlog_raw\tgps_raw\t\tsystem status\tnormal 2 27.900000 0 0\trobot status\t120.478815\t125.601217\t7.971200\t0.419011\t-1.042839\t-176.916783\t0.295000\t0.000000\n\t\n15:46:26.1\tlog_raw\tgps_raw\t\tsystem status\tnormal 2 27.900000 0 0\trobot status\t120.330401\t125.606481\t7.967500\t0.504223\t-1.248661\t-177.001637\t0.300000\t-0.003000
